vi "set reservation info.vi"(0 "Section Ptr":T1 format="%.0x", 5 "channel type":T2, 7 "datatype":variant, 9 "Pattern":string, 11 "error in (no error)":errorcluster) -> (4 "Item Ref out":T1 format="%.0x", 15 "error out":errorcluster)   [LabVIEW 2016, in "FPGA RM System Definition API.lvlib"]
uses:
  <vilib>/NI Veristand/Custom Device API/Custom Device Item Ref.ctl
  Channel Type.ctl
  <vilib>/NI Veristand/Custom Device API/Set Item Property (Variant).vi
  <vilib>/NI Veristand/Custom Device API/Set Item Property (U16).vi
  <vilib>/NI Veristand/Custom Device API/Set Item Property (String).vi
  FPGA RM System Definition API.lvlib
  <vilib>/NI VeriStand/Custom Device API/Custom Device API.lvlib
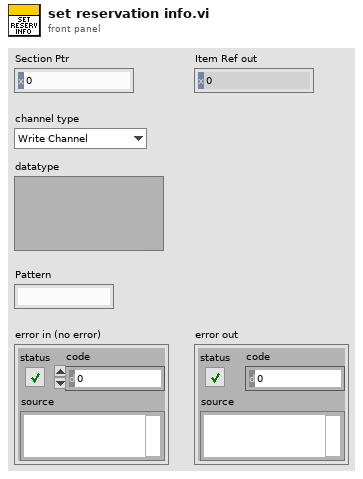
[diagram p1: front panel]
types:
  T1 = typedef "Custom Device API.lvlib/Custom Device Item Ref.ctl" = u64
  T2 = typedef "FPGA RM System Definition API.lvlib/Channel Type.ctl" = enum16{"Write Channel", "Read Channel", "Write Waveform", "Read Waveform"}
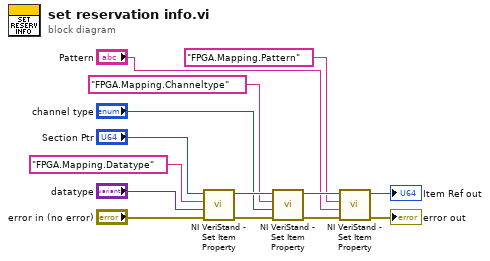
[diagram p0: block diagram]
diagram:
  n1 = call-poly <vilib>:"NI VeriStand - Set Item Property.vi"("error in (no error)"="error in (no error)", "Value"="datatype", "Property Name"="FPGA.Mapping.Datatype", "Item Ref in"="Section Ptr") -> ("error out"=w7:errorcluster, "Item Ref out"=w11:T1)  [unwired: 5 in, 1 out]
  n2 = call-poly <vilib>:"NI VeriStand - Set Item Property.vi"("error in (no error)"=w7, "Value"="channel type", "Property Name"="FPGA.Mapping.Channeltype", "Item Ref in"=w11) -> ("error out"=w6:errorcluster, "Item Ref out"=w4:T1)  [unwired: 5 in, 1 out]
  n3 = call-poly <vilib>:"NI VeriStand - Set Item Property.vi"("error in (no error)"=w6, "Value"="Pattern", "Property Name"="FPGA.Mapping.Pattern", "Item Ref in"=w4) -> ("error out"=→"error out":errorcluster, "Item Ref out"=→"Item Ref out":T1)  [unwired: 5 in, 1 out]
